vi "Send-priority-message.vi"(8 "error in (no error)":errorcluster, 9 "Receivers":string[](array[string]), 10 "Message":refnum<class "Message.lvclass">, 11 "Client in":T1) -> (0 "error out":errorcluster, 3 "Client out":T1)   [LabVIEW 2013, in "PowderDeposition.lvlib" / "PD-Client.lvclass"]
doc: "Send a message to the specified list of receivers.\nThe message is added to the front of the server message queue and will be treated with priority.\nThe message needs to be created beforehand, either manually or through the 'Create-message' function and any specific contents need to be pre-configured. This function takes care of the sender and time information.\nThe receivers must be provided as an array. Each receiver entry can be composed in two ways: either '<module type>' to send to all active clients of the specified type, or '<module type><module ID>' to send to a specific client. Optionally the special client types 'All' or 'Server' can be used to send the message to all active clients (server excluded) or to the server, respectively."
uses:
  PD-Client.lvclass
  Object-reference.ctl
  SA-SLMAPI/Sources/Message.lvclass
  PD-Client.lvclass/PD-Client.ctl
  Main/PD-Main.lvclass
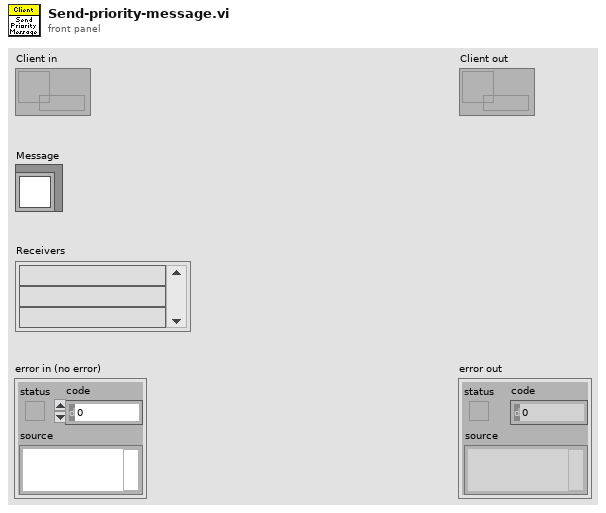
[diagram p1: front panel]
types:
  T1 = typedef "PowderDeposition.lvlib/PD-Client.lvclass/Object-reference.ctl" = refnum<data-value>
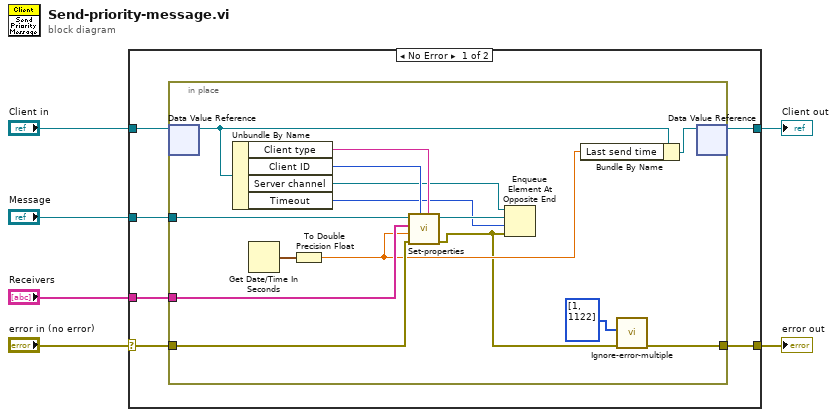
[diagram p0: block diagram]
diagram:
  n1 = case shown="No Error" "error in (no error)" {
    selector: "error in (no error)" -> [w8 w29]
    tunnel: [w7 w29] -> w5
    tunnel: [w9 w28] -> w3
    tunnel: "Client in" -> [w10 w28]
    tunnel: "Message" -> [w12 _]
    tunnel: "Receivers" -> [w11 _]
    frame No Error {
      n2 = in-place {
        in-place-border: w12 -> [w27]
        in-place-border: w11 -> [w26]
        in-place-border: w8 -> [w24]
        in-place-border: [w13] -> w7
        n3 = in-place-dvr #1(w10) -> (w18:refnum<class "PD-Client.lvclass">)  [unwired: 1 out]
        n4 = Unbundle By Name(w18) -> ("Client type"=w22:string, "Client ID"=w23:i32, "Server channel"=w19:refnum<queue>, "Timeout"=w20:i32)
        n5 = Get Date/Time In Seconds() -> (seconds since 1Jan1904=w25:timestamp)
        n6 = To Double Precision Float(number=w25) -> (double precision float=w16:dbl)
        n7 = call-dynamic "Set-properties.vi"("Sender type"=w22, "Sender ID"=w23, "error in (no error)"=w24, "Send time"=w16, "Receivers"=w26, "Message in"=w27) -> ("error out"=w14:errorcluster, "Message out"=w21:refnum<class "Message.lvclass">)  [unwired: 4 in]
        n8 = Enqueue Element At Opposite End(queue=w19, element=w21, timeout in ms (-1)=w20, error in (no error)=w14) -> ()  [unwired: 3 out]
        n9 = Bundle By Name(cluster=w18, "Last send time"=w16) -> (w17:refnum<class "PD-Client.lvclass">)
        n10 = call "Ignore-error-multiple.vi"("error in (no error)"=w14, "Errors to ignore (1)"=i32[] [1, 1122]) -> ("error out"=w13:errorcluster)  [unwired: 9 in]
        n11 = in-place-dvr #1(w17) -> (w9:T1)  [unwired: 1 out]
      }
    }
    frame Error {
    }
  }
  "error out" <- w5
  "Client out" <- w3
